vi "ContourFilled_Manual.vi"(4 "Properties":T1={"Colormap"={"Map"=enum."Automatic", "Value Min"=nan, "Value Max"=nan, "Scaling"=enum."Default", "Reverse"=FALSE}, "Display"={"Alpha"=nan, "Z Order"=nan}}, 5 "Levels":dbl[](array[numeric]), 7 "Z Data":dbl[][](array[numeric]), 8 "error in (no error)":errorcluster, 9 "Y Coordinates":dbl[](array[numeric]), 10 "X Coordinates":dbl[](array[numeric]), 11 "Plot ID":T6 format="%x") -> (0 "error out":errorcluster, 3 "Plot ID Out":T6 format="%x")   [LabVIEW 2013, in "Advanced Plotting Toolkit.lvlib"]
doc: "Generate a filled contour plot, using explicitly specified contour levels.\n\nNote this VI does the filled regions only; use Contour.vi for lines."
uses:
  Advanced Plotting Toolkit.lvlib
  typedefs/PlotID.ctl
  ContourFilledProperties.ctl
  properties/Colormap.ctl
  properties/Colormap_Map.ctl
  properties/Colormap_Scaling.ctl
  properties/Display.ctl
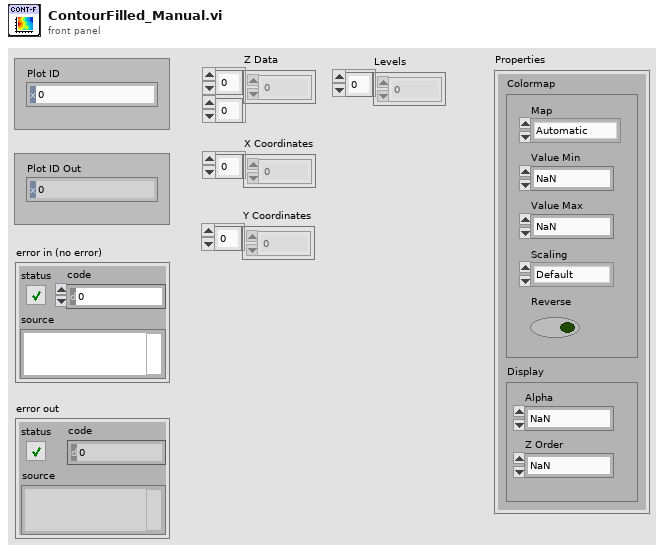
[diagram p1: front panel]
types:
  T1 = typedef "Advanced Plotting Toolkit.lvlib/ContourFilledProperties.ctl" = cluster{"Colormap":T2, "Display":T5}
  T2 = typedef "Advanced Plotting Toolkit.lvlib/Colormap.ctl" = cluster{"Map":T3, "Value Min":dbl, "Value Max":dbl, "Scaling":T4, "Reverse":bool}
  T3 = typedef "Advanced Plotting Toolkit.lvlib/Colormap_Map.ctl" = enum16{"Automatic", "Rainbow", "Hot and Cold", "White-Black", "White-Blue", "White-Green", "White-Red", "Fire", "Water", "Earth", "Air", "Pastel", "Banded", "Stepped"}
  T4 = typedef "Advanced Plotting Toolkit.lvlib/Colormap_Scaling.ctl" = enum16{"Default"}
  T5 = typedef "Advanced Plotting Toolkit.lvlib/Display.ctl" = cluster{"Alpha":dbl, "Z Order":dbl}
  T6 = typedef "Advanced Plotting Toolkit.lvlib/PlotID.ctl" = i32
  T7 = typedef "Advanced Plotting Toolkit.lvlib/KeyValue.ctl" = cluster{"Key":string, "Value":string}
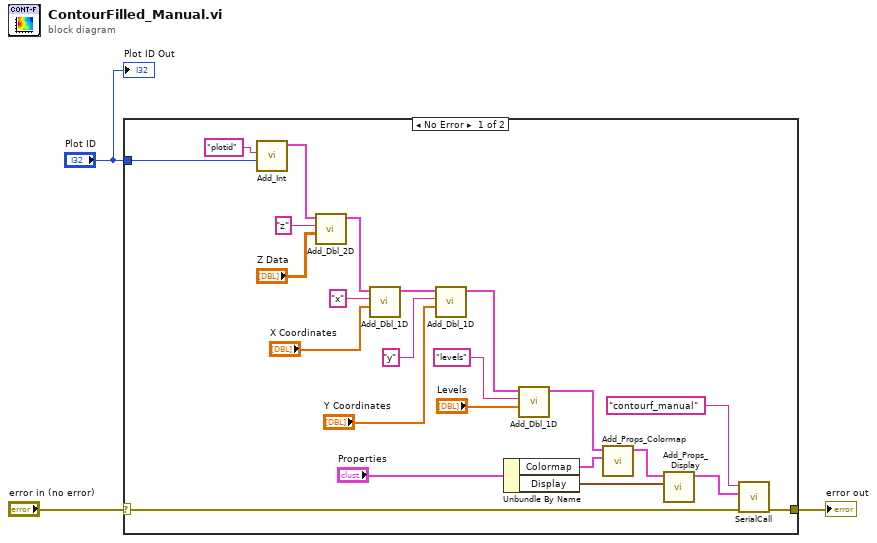
[diagram p0: block diagram]
diagram:
  n1 = case shown="No Error" "error in (no error)" {
    selector: "error in (no error)" -> [w17 w27]
    tunnel: "Plot ID" -> [w15 _]
    tunnel: [w16 w27] -> w1
    frame No Error {
      n2 = call "Add_Int.vi"("Value"=w15, "Key"="plotid") -> ("Keyword Array Out"=w22:T7[])  [unwired: 9 in]
      n3 = call "Add_Dbl_2D.vi"("Value"="Z Data", "Key"="z", "Keyword Array"=w22) -> ("Keyword Array Out"=w21:T7[])  [unwired: 8 in]
      n4 = call "Add_Dbl_1D.vi"("Value"="X Coordinates", "Key"="x", "Keyword Array"=w21) -> ("Keyword Array Out"=w20:T7[])  [unwired: 8 in]
      n5 = call "Add_Dbl_1D.vi"("Value"="Y Coordinates", "Key"="y", "Keyword Array"=w20) -> ("Keyword Array Out"=w7:T7[])  [unwired: 8 in]
      n6 = Unbundle By Name("Properties") -> ("Colormap"=w10:T2, "Display"=w8:T5)
      n7 = call "Add_Dbl_1D.vi"("Value"="Levels", "Key"="levels", "Keyword Array"=w7) -> ("Keyword Array Out"=w4:T7[])  [unwired: 8 in]
      n8 = call "Add_Props_Colormap.vi"("Colormap"=w10, "Keyword Array"=w4) -> ("Keyword Array Out"=w9:T7[])  [unwired: 9 in]
      n9 = call "Add_Props_Display.vi"("Display"=w8, "Keyword Array"=w9) -> ("Keyword Array Out"=w11:T7[])  [unwired: 9 in]
      n10 = call "SerialCall.vi"("error in (no error)"=w17, "data"=w11, "Resource"="contourf_manual") -> ("error out"=w16:errorcluster)  [unwired: 7 in, 1 out]
    }
    frame Error {
    }
  }
  "error out" <- w1
  "Plot ID Out" <- "Plot ID"
